vi "Config Control Mode.vi"(0 "VISA resource name":refnum<visa-resource-name>, 1 "Control Mode (0: Manual PID)":u16(ring) items=["Manual PID", "Zone", "Open Loop"], 2 "Setpoint Units (0: Kelvin)":u16(ring) items=["Kelvin", "Celsius", "Sensor Units"], 5 "Loop (0: 1)":u16(ring) items=["1", "2"], 7 "Input to \nControl From (0: A)":u16(ring) items=["A", "B", "C", "D"], 9 "Control (F: Control Off)":bool, 11 "error in (no error)":errorcluster, 12 "Powerup Enable (F: Disable)":bool) -> (4 "VISA resource name out":refnum<visa-resource-name>, 15 "error out":errorcluster)   [LabVIEW 2019, in "Lake Shore Cryotronics 340.lvlib"]
doc: "This VI selects a control loop's mode and configures the parameters of a control loop."
uses:
  Lake Shore Cryotronics 340.lvlib
panel:
  # "Control On\nControl Off"
  # "Enable\nDisable"
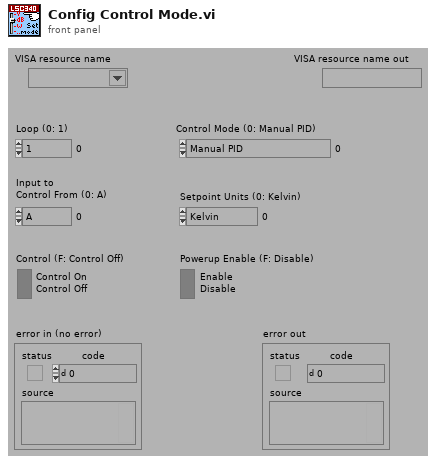
[diagram p1: front panel]
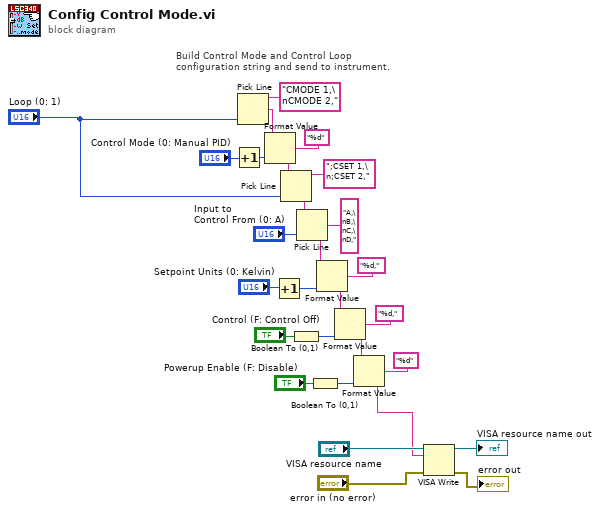
[diagram p0: block diagram]
diagram:
  # "Build Control Mode and Control Loop\nconfiguration string and send to instrument."
  n1 = Increment(x="Control Mode (0: Manual PID)") -> (x+1=w8:u16)
  n2 = Pick Line(multi-line string="CMODE 1,\nCMODE 2,", line index="Loop (0: 1)") -> (output string=w17:string)  [unwired: 1 in]
  n3 = Format Value(string ("")=w17, format string="%d", value (0)=w8) -> (output string=w16:string)
  n4 = Increment(x="Setpoint Units (0: Kelvin)") -> (x+1=w23:u16)
  n5 = Pick Line(string ("")=w16, multi-line string=";CSET 1,\n;CSET 2,", line index="Loop (0: 1)") -> (output string=w13:string)
  n6 = Boolean To (0,1)(Boolean="Control (F: Control Off)") -> (0, 1=w25:i16)
  n7 = Pick Line(string ("")=w13, multi-line string="A,\nB,\nC,\nD,", line index="Input to \nControl From (0: A)") -> (output string=w12:string)
  n8 = Boolean To (0,1)(Boolean="Powerup Enable (F: Disable)") -> (0, 1=w21:i16)
  n9 = Format Value(string ("")=w12, format string="%d,", value (0)=w23) -> (output string=w10:string)
  n10 = Format Value(string ("")=w10, format string="%d,", value (0)=w25) -> (output string=w9:string)
  n11 = Format Value(string ("")=w9, format string="%d", value (0)=w21) -> (output string=w1:string)
  n12 = VISA Write(VISA resource name="VISA resource name", write buffer=w1, error in (no error)="error in (no error)") -> (VISA resource name out=→"VISA resource name out":refnum<visa-resource-name>, error out=→"error out":errorcluster)  [unwired: 1 out]
